vi "FindMatchingRules.vi"(8 "error in (no error)":errorcluster, 9 "Item to match":refnum<class "ILabVIEWItem.lvclass">, 11 "CRuleList in":refnum<class "CRuleList.lvclass">) -> (0 "error out":errorcluster, 1 "Matching rules":refnum<class "IDependencyItemRule.lvclass">[](array[class]), 2 "rules found?":bool, 3 "CRuleList out":refnum<class "CRuleList.lvclass">)   [LabVIEW 2020, in "DependencyInspection.lvlib" / "CRuleList.lvclass"]
uses:
  CRuleList.lvclass
  obj/Addons/LabVIEWObjectInterfaces.lvlibp/LabVIEWObjectInterfaces/ILabVIEWItem/ILabVIEWItem.lvclass
  obj/Addons/LabVIEWObjectInterfaces.lvlibp/LabVIEWObjectInterfaces/IDependencyItemRule/IDependencyItemRule.lvclass
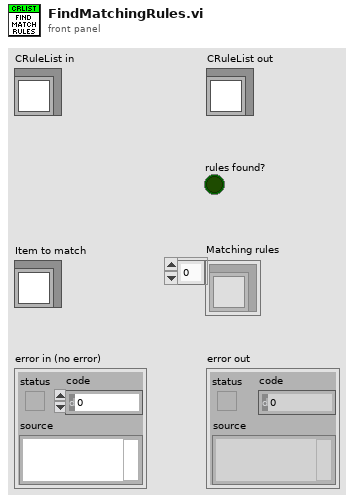
[diagram p1: front panel]
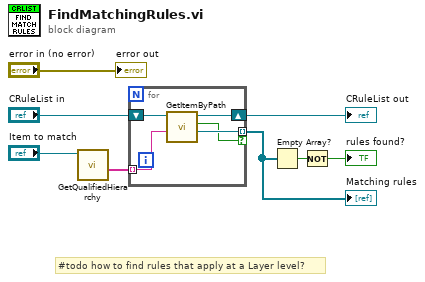
[diagram p0: block diagram]
diagram:
  # "#todo how to find rules that apply at a Layer level?"
  n1 = call-dynamic "GetQualifiedHierarchy.vi"("ILabVIEWItem in"="Item to match") -> ("Qualified hierarchy"=w1:string[])  [unwired: 8 in, 2 out]
  n2 = for {
    shift-right: [w12] -> w5
    shift-left: "CRuleList in" -> [w13]
    tunnel: w1 -> [w11] mode=indexing
    tunnel: [w10] -> w3 mode=indexing if=w9
    n3 = call-dynamic "GetItemByPath.vi"("Path"=w11, "CRuleList in"=w13) -> ("IDependencyItemRule"=w10:refnum<class "IDependencyItemRule.lvclass">, "key found?"=w9:bool, "CRuleList out"=w12:refnum<class "CRuleList.lvclass">)  [unwired: 6 in, 1 out]
  }
  "CRuleList out" <- w5
  "Matching rules" <- w3
  n4 = Empty Array?(array=w3) -> (empty?=w2:bool)
  n5 = Not(x=w2) -> (.not. x?=→"rules found?":bool)
  "error out" <- "error in (no error)"
